vi "Generate Unexpected Number Of Channels Error.vi"(8 "error in (no error)":errorcluster, 9 "Actual Channel Names":string[](array[string]), 10 "Actual Number of Channels":i32, 11 "Expected Number of Channels":i32) -> (0 "error out":errorcluster)   [LabVIEW 2020, in "Error Provider API.lvlib"]
uses:
  <vilib>/NI VeriStand/Error Provider API/Error Provider API.lvlib
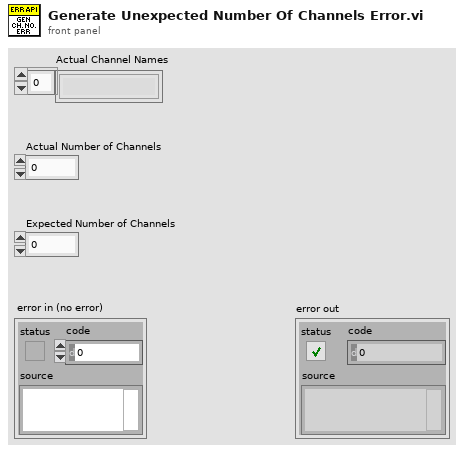
[diagram p1: front panel]
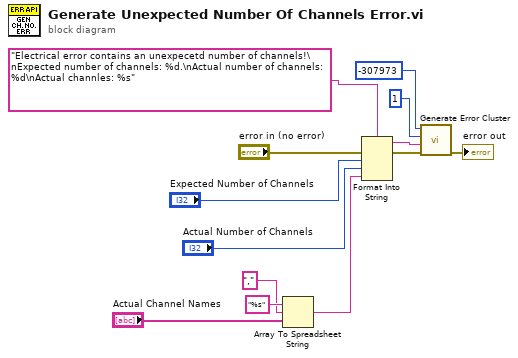
[diagram p0: block diagram]
diagram:
  n1 = Array To Spreadsheet String(delimiter (Tab)=",", array="Actual Channel Names", 3:"%s" ("format string")) -> (spreadsheet string=w7:string)
  n2 = Format Into String(format string="Electrical error contains an unexpecetd number of channels!\nExpected number of channels: %d.\nActual number of channels: %d\nActual channles: %s", error in="error in (no error)", "Expected Number of Channels", "Actual Number of Channels", w7) -> (resulting string=w4:string, error out=w5:errorcluster)  [unwired: 1 in]
  n3 = call <vilib>:"Generate Error Cluster.vi"("error in (no error)"=w5, "Additional Message"=w4, "CallChainLvl (-1 => No call chain)"=1, "Code"=-307973) -> ("error out"=→"error out":errorcluster)  [unwired: 7 in]
